vi "Set Axis Cam Exposure.vi"(9 "Exposure Value":i32) -> ()   [LabVIEW 2013]
uses:
  Common Code/Change Detect Int.vi
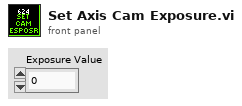
[diagram p1: front panel]
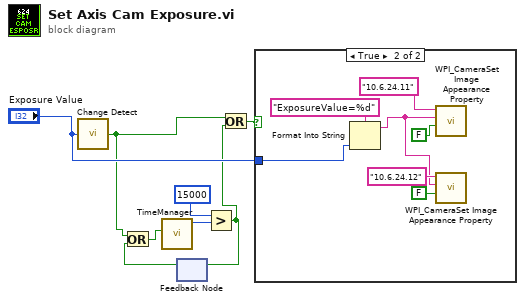
[diagram p0: block diagram]
diagram:
  n1 = call-poly "Change Detect.vi"("In"="Exposure Value") -> ("Changed?"=w2:bool)
  n2 = feedback #1() -> (w4:bool)  [unwired: 1 in]
  n3 = Or(x=w2, y=w4) -> (x .or. y?=w5:bool)
  n4 = call "TimeManager.vi"("Reset?"=w5) -> ("Time Since Reset"=w7:u32)  [unwired: 9 in, 1 out]
  n5 = Greater?(x=u32 15000, y=w7) -> (0:w1:bool)
  n6 = feedback-in #1(w1) -> ()
  n7 = Or(x=w2, y=w1) -> (x .or. y?=w3:bool)
  n8 = case shown="True" w3 {
    tunnel: "Exposure Value" -> [_ w12]
    frame False {
    }
    frame True {
      n9 = Format Into String(format string="ExposureValue=%d", w12) -> (resulting string=w10:string)  [unwired: 2 in, 1 out]
      n10 = call <vilib>:"WPI_CameraSet Image Appearance Property.vi"("Appearance"=FALSE, "Prop String"=w10, "address"="10.6.24.11") -> ()  [unwired: 8 in, 1 out]
      n11 = call <vilib>:"WPI_CameraSet Image Appearance Property.vi"("Appearance"=FALSE, "Prop String"=w10, "address"="10.6.24.12") -> ()  [unwired: 8 in, 1 out]
    }
  }
